vi "CS SQL Server.send command.vi"(3 "error in (no error)":errorcluster, 4 "SQL Command":string, 5 "Data Source":string) -> (0 "error out":errorcluster, 1 "Class":string, 2 "query results":string[][](table))   [LabVIEW 2014, in "CS SQL Server.lvlib"]
doc: "This VI executes a SQL statement and may retrieves data (tested with MS Access).\n\nLicense Agreement:\n\nCopyright (C)\nGesellschaft für Schwerionenforschung, GSI\nPlanckstr. 1\n64291 Darmstadt\nGermany\n\nContact: A.Schwinn@gsi.de \n\nThis program is free software; you can redistribute it and/or modify it under the terms of the \nGNU General Public License as published by the Free Software Foundation; either version 2 of the license, or (at your option) any later version.\n\nThis program is distributed in the hope that it will be useful, but WITHOUT ANY WARRANTY; without even the implied warranty of MERCHANTABILITY or FITNESS FOR A PARTICULAR PURPOSE. See the GNU General License for more details (http://www.gnu.org).\n\nGesellschaft für Schwerionenforschung, GSI\nPlanckstr. 1, 64291 Darmstadt, Germany\nFor all questions and ideas contact: M.Richter@gsi.de, K.Poppensieker, H.Brand@gsi.de or D.Beck@gsi.de.\nLast update: 24-OCT-2008"
uses:
  CS SQL Server.lvlib
  <vilib>/addons/database/Recordset.llb/Rec Destroy - Connection.vi
  <vilib>/addons/database/Recordset.llb/Rec Fetch Recordset Data (R).vi
  <vilib>/addons/database/Connection.llb/Conn Execute.vi
  <vilib>/addons/database/Connection.llb/DB Tools Open Connec (String).vi
  <vilib>/addons/database/_DB Variant To Data/Database Variant To Data.xnode
  <vilib>/addons/database/NI_Database_API.lvlib
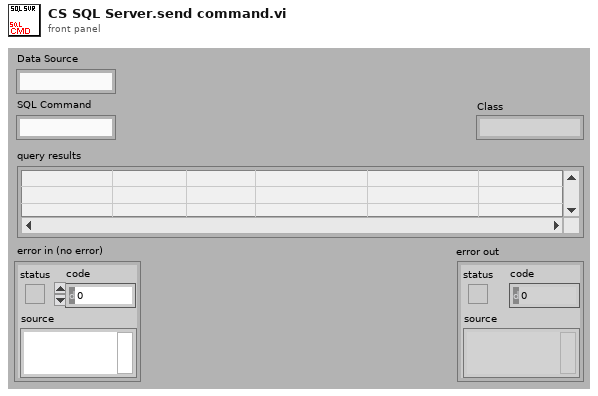
[diagram p1: front panel]
types:
  T1 = typedef "NI_Database_API.lvlib/Conn ObjectReference.ctl" = refnum<k1>
  T2 = typedef "NI_Database_API.lvlib/Rec ObjectReference.ctl" = refnum<k1>
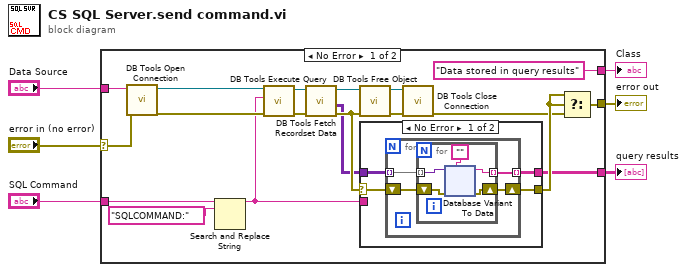
[diagram p0: block diagram]
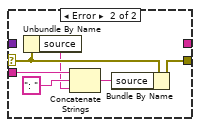
[diagram p2: hidden frame]
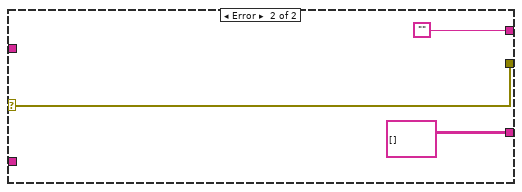
[diagram p3: hidden frame]
diagram:
  n1 = case shown="No Error" "error in (no error)" {
    selector: "error in (no error)" -> [w25 w79]
    tunnel: "Data Source" -> [w9 _]
    tunnel: "SQL Command" -> [w22 _]
    tunnel: [w7 string[][] []] -> w4
    tunnel: [w18 w79] -> w3
    tunnel: ["Data stored in query results" ""] -> w1
    frame No Error {
      n2 = call-poly <vilib>:"DB Tools Open Connection.vi"("error in (no error)"=w25, "connection information"=w9) -> ("error out"=w23:errorcluster, "connection reference"=w24:T1)  [unwired: 6 in]
      n3 = Search and Replace String(input string=w22, search string="SQLCOMMAND:") -> (result string=w19:string)  [unwired: 6 in, 3 out]
      n4 = call-poly <vilib>:"DB Tools Execute Query.vi"("error in (no error)"=w23, "SQL query"=w19, "connection reference"=w24) -> ("error out"=w15:errorcluster, "recordset reference"=w14:T2)  [unwired: 5 in]
      n5 = call-poly <vilib>:"DB Tools Fetch Recordset Data.vi"("error in (no error)"=w15, "recordset reference"=w14) -> ("error out"=w10:errorcluster, "recordset data"=w8:variant[][], "recordset reference out"=w13:T2)  [unwired: 3 in]
      n6 = call-poly <vilib>:"DB Tools Free Object.vi"("error in (no error)"=w10, "recordset reference"=w13) -> ("error out"=w12:errorcluster, "connection reference"=w11:T1)  [unwired: 8 in]
      n7 = case shown="No Error" w10 {
        selector: w10 -> [w28 w73]
        tunnel: [w26 w71] -> w17
        tunnel: w19 -> [_ w74]
        tunnel: w8 -> [w29 _]
        tunnel: [w27 _] -> w7
        frame No Error {
          n8 = for {
            tunnel: w29 -> [w33] mode=indexing
            shift-right: [w31] -> w26
            shift-left: w28 -> [w32]
            tunnel: [w30] -> w27 mode=indexing
            n9 = for {
              tunnel: w33 -> [w38] mode=indexing
              shift-right: [w36] -> w31
              shift-left: w32 -> [w37]
              tunnel: [w34] -> w30 mode=indexing
              n10 = xnode "Database Variant To Data"("database variant"=w38, "error in (no error)"=w37, "type"="") -> ("data"=w34:string, "error out"=w36:errorcluster)
            }
          }
        }
        frame Error {
          n11 = Unbundle By Name(w73) -> ("source"=w72:string)
          n12 = Concatenate Strings(w74, ": " ("string"), w72) -> (w76:string)
          n13 = Bundle By Name(cluster=w73, "source"=w76) -> (w71:errorcluster)
        }
      }
      n14 = call <vilib>:"DB Tools Close Connection.vi"("error in (no error)"=w12, "connection reference"=w11) -> ("error out"=w16:errorcluster)  [unwired: 5 in]
      n15 = Select(t=w17, s=w17, f=w16) -> (s? t:f=w18:errorcluster)
    }
    frame Error {
    }
  }
  "query results" <- w4
  "error out" <- w3
  "Class" <- w1
